vi "Send Configure Number of Envelopes [MmW].vi"(7 "Message Priority (Normal)":T1=enum."Normal", 8 "error in (no error)":errorcluster, 10 "number of envelopes (8)":i32=8, 11 "Message Enqueuer":refnum<class "Message Enqueuer.lvclass">) -> (0 "error out":errorcluster, 3 "Message Enqueuer out":refnum<class "Message Enqueuer.lvclass">)   [LabVIEW 2015, in "CS++Scope.lvlib" / "Configure Number of Envelopes [MmW] Msg.lvclass"]
doc: "Sends the <B>CS++Scope.lvlib:Configure Number of Envelopes [MmW] Msg.lvclass</B> message.\n\n<B>CS++Scope.lvlib:CS++Scope.lvclass:Configure Number of Envelopes [MmW].vi</B> Description:\n\nWhen you set the acquisition type to IVISCOPE_VAL_ENVELOPE, the oscilloscope acquires multiple waveforms. After each waveform acquisition, the oscilloscope keeps the minimum and maximum values it finds for each element in the waveform record. This VI configures the number of waveforms the oscilloscope acquires and analyzes to create the minimum and maximum waveforms. After the oscilloscope acquires as many waveforms as you specify, it returns to the idle state."
uses:
  Configure Number of Envelopes [MmW] Msg.lvclass
  <vilib>/ActorFramework/Message Enqueuer/Message Enqueuer.lvclass
  <vilib>/ActorFramework/Message Enqueuer/Message Priority.ctl
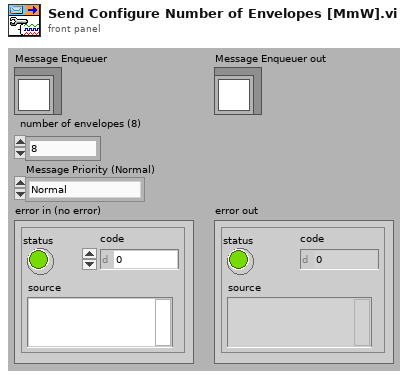
[diagram p1: front panel]
types:
  T1 = typedef "Actor Framework.lvlib/Message Enqueuer.lvclass/Message Priority.ctl" = enum16{"Low", "Normal", "High"}
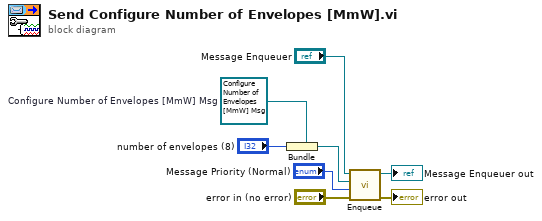
[diagram p0: block diagram]
diagram:
  w2 = refnum<class "Configure Number of Envelopes [MmW] Msg.lvclass"> refnum  # Configure Number of Envelopes [MmW] Msg
  n1 = Bundle(cluster=w2, "number of envelopes (8)") -> (w5:refnum<class "Configure Number of Envelopes [MmW] Msg.lvclass">)
  n2 = call <vilib>:"Enqueue.vi"("error in (no error)"="error in (no error)", "Message Priority (Normal)"="Message Priority (Normal)", "Message"=w5, "Message Enqueuer in"="Message Enqueuer") -> ("error out"=→"error out":errorcluster, "Message Enqueuer out"=→"Message Enqueuer out":refnum<class "Message Enqueuer.lvclass">)  [unwired: 6 in]
